vi "HFRR ADV v05.vi"() -> ()   [LabVIEW 2025] (continued)
                n2416 = Wait (ms)(milliseconds to wait=u32 200) -> ()  [unwired: 1 out]
              }
            }
            n2417 = local read "Com Port 3"() -> (w3502:refnum<visa-resource-name>)
            n2418 = local read "Humidity Str Rec"() -> (w3504:string)
            n2419 = Not Equal?(x="Set Rh", y=w3526) -> (x != y?=w3531:bool)
            n2420 = Number To Decimal String(number="Set Rh") -> (decimal integer string=w3529:string)  [unwired: 1 in]
            n2421 = Not Equal?(x=w3502, y=w3501) -> (x != y?=w3497:bool)
            n2422 = Concatenate Strings("#setPoint00" ("string"), w3529) -> (w3530:string)
            n2423 = case shown="False" w3531 {
              tunnel: w3530 -> [_ w3550]
              frame False {
                n2424 = local read "Humidity"() -> (w3547:bool)
                n2425 = case shown="True" w3547 {
                  frame False {
                    n2426 = local write "Humidity Str Send"("stop" ("Humidity Str Send")) -> ()
                  }
                  frame True {
                    n2427 = local write "Humidity Str Send"("start" ("Humidity Str Send")) -> ()
                  }
                }
              }
              frame True {
                n2428 = local write "Humidity Str Send"(w3550) -> ()
              }
            }
            n2429 = Or(x=w3497, y="Re-Initialise") -> (x .or. y?=w3496:bool)
            n2430 = String Subset(string=w3504, offset (0)=7) -> (substring=w3519:string)  [unwired: 1 in]
            n2431 = Match Pattern(string=w3504, regular expression="?") -> (offset past match=w3522:i32)  [unwired: 1 in, 3 out]
            n2432 = Match Pattern(string=w3504, regular expression="v") -> (offset past match=w3525:i32)  [unwired: 1 in, 3 out]
            n2433 = case shown="True" w3496 {
              tunnel: w3499 -> [w3536 _]
              tunnel: [w3536 errorcluster {"status"=TRUE, "code"=0, "source"="Init"} ("error out")] -> w3498
              frame False {
              }
              frame True {
              }
            }
            n2434 = Equal?(x=w3522, y=-1) -> (x = y?=w3506:bool)
            n2435 = Match Pattern(string=w3519, regular expression="g") -> (after substring=w3520:string, offset past match=w3511:i32)  [unwired: 1 in, 2 out]
            n2436 = Match Pattern(string=w3519, regular expression="y") -> (after substring=w3518:string, offset past match=w3512:i32)  [unwired: 1 in, 2 out]
            n2437 = Greater?(x=w3512, y=w3511) -> (0:w3517:bool)
            n2438 = Greater Or Equal To 0?(x=w3512) -> (x >= 0?=w3509:bool)
            n2439 = Greater Or Equal To 0?(x=w3511) -> (x >= 0?=w3510:bool)
            n2440 = Or(x=w3509, y=w3510) -> (x .or. y?=w3508:bool)
            n2441 = Greater Or Equal To 0?(x=w3525) -> (x >= 0?=w3507:bool)
            n2442 = Select(t=w3518, s=w3517, f=w3520) -> (s? t:f=w3513:string)
            n2443 = case shown="Error" w3498 {
              selector: w3498 -> [w3563 w3609]
              tunnel: [w3561 w3602] -> w3535
              tunnel: w3501 -> [w3564 w3608]
              tunnel: [w3562 w3611] -> w3534
              tunnel: w3532 -> [w3551 w3610]
              tunnel: [w3558 w3610] -> w3533
              frame No Error {
                n2444 = call "Elapsed Time7"() -> ("Time has Elapsed"=w3557:bool)  [unwired: 12 in, 7 out]
                n2445 = Not Equal?(x="Humidity Str Send", y=w3551) -> (x != y?=w3553:bool)
                n2446 = Or(x=w3553, y=w3557) -> (x .or. y?=w3556:bool)
                n2447 = Select(t="Humidity Str Send", s=w3553, f="vals" ("regular expression")) -> (s? t:f=w3552:string)
                n2448 = Or(x=w3556, y="Send") -> (x .or. y?=w3560:bool)
                n2449 = case shown="True" w3560 {
                  tunnel: [w3567 w3572] -> w3561
                  tunnel: w3564 -> [w3566 w3580]
                  tunnel: w3563 -> [w3567 w3579]
                  tunnel: [w3566 w3573] -> w3562
                  tunnel: w3552 -> [_ w3578]
                  tunnel: [w3565 w3569] -> w3558
                  tunnel: "Humidity Str Send" -> [_ w3570]
                  tunnel: w3553 -> [_ w3571]
                  tunnel: w3551 -> [w3565 w3568]
                  frame False {
                  }
                  frame True {
                    n2450 = flat-sequence {
                      tunnel: w3580 -> [w3588]
                      tunnel: w3579 -> [w3587]
                      tunnel: w3578 -> [w3584]
                      tunnel: [w3586] -> w3577
                      tunnel: [w3585] -> w3576
                      tunnel: w3577 -> [w3591]
                      tunnel: w3576 -> [w3590]
                      tunnel: [w3591] -> w3575
                      tunnel: [w3590] -> w3574
                      tunnel: w3575 -> [w3598]
                      tunnel: w3574 -> [w3597]
                      tunnel: [w3596] -> w3573
                      tunnel: [w3595] -> w3572
                      frame #0 {
                        n2451 = local write "Ser Led"(TRUE ("Boolean 4")) -> ()
                        n2452 = Concatenate Strings(w3584, "\r") -> (w3583:string)
                        n2453 = VISA Write(VISA resource name=w3588, write buffer=w3583, error in (no error)=w3587) -> (VISA resource name out=w3586:refnum<visa-resource-name>, error out=w3585:errorcluster)  [unwired: 1 out]
                      }
                      frame #1 {
                        n2454 = Wait (ms)(milliseconds to wait="wait") -> ()  [unwired: 1 out]
                      }
                      frame #2 {
                        w3593 = FALSE ("Send")
                        n2455 = property class="Instr"(reference=w3598, error in=w3597) -> (reference out=w3599:refnum<visa-resource-name>, error out=w3600:errorcluster, "Serial Settings:Number of Bytes at Serial Port"=w3592:u32)
                        "Humidity 2" <- w3592
                        n2456 = local write "Send"(w3593) -> ()
                        n2457 = local write "Ser Led"(w3593) -> ()
                        n2458 = VISA Read(VISA resource name=w3599, byte count=w3592, error in (no error)=w3600) -> (VISA resource name out=w3596:refnum<visa-resource-name>, read buffer=→"Humidity Str Rec":string, error out=w3595:errorcluster)  [unwired: 1 out]
                      }
                    }
                    n2459 = Select(t=w3570, s=w3571, f=w3568) -> (s? t:f=w3569:string)
                  }
                }
              }
              frame Error {
                w3616 = u16 0 items=["None"=0, "XON/XOFF"=1, "RTS/CTS"=2, "DTR/DSR"=4] ("flow control")
                w3612 = u16 0 items=["None", "Odd", "Even", "Mark", "Space"] ("parity")
                w3615 = u16 10 items=["1.0"=10, "1.5"=15, "2.0"=20] ("stop bits")
                n2460 = VISA Close(VISA resource name=w3608, error in (no error)=w3609) -> (error out=w3607:errorcluster)
                n2461 = local write "humid"("" ("humid")) -> ()
                n2462 = local write "Humidity Str Rec"("" ("Humidity Str Rec")) -> ()
                n2463 = call <vilib>:"Clear Errors.vi"("error in (no error)"=w3607) -> ("error out"=w3606:errorcluster)  [unwired: 5 in, 1 out]
                n2464 = local read "Com Port 3"() -> (w3605:refnum<visa-resource-name>)
                n2465 = call-poly "VISA Configure Serial Port"("VISA resource name"=w3605, "timeout (10sec)"=u32 1000, "termination char\n(0xA = '\\n' = LF)"=u8 10 ("termination char\n(0xA = '\\n' = LF)"), "Enable Termination\nChar (T)"=FALSE ("Enable Termination Char (T)"), "baud rate (9600)"="Humidity BaudRate", "data bits (8)"=u16 8 ("data bits"), "parity (0:none)"=w3612, "error in (no error)"=w3606, "stop bits (10: 1 bit)"=w3615, "flow control (0:none)"=w3616) -> ("VISA resource name out"=w3611:refnum<visa-resource-name>, "error out"=w3602:errorcluster)  [unwired: 4 in]
              }
            }
            n2466 = Compound Arithmetic op=AND(w3507, w3506, w3508) -> (w3505:bool)
            n2467 = case shown="True" w3505 {
              tunnel: w3504 -> [_ _]
              tunnel: w3513 -> [_ w3543]
              frame False {
              }
              frame True {
                w3541 = " " ("regular expression")
                n2468 = Match Pattern(string=w3543, regular expression=" ") -> (after substring=w3545:string)  [unwired: 1 in, 3 out]
                n2469 = Match Pattern(string=w3545, regular expression=w3541) -> (before substring=→"humid":string, after substring=w3542:string)  [unwired: 1 in, 2 out]
                n2470 = Match Pattern(string=w3542, regular expression=w3541) -> (before substring=→"temp_@Rh sensor":string)  [unwired: 1 in, 3 out]
              }
            }
            n2471 = local read "Quit"() -> (w3494:bool)
          }
          n2472 = VISA Close(VISA resource name=w3490, error in (no error)=w3491) -> (error out=w3487:errorcluster)
          n2473 = call <vilib>:"Clear Errors.vi"("error in (no error)"=w3487) -> ()  [unwired: 5 in, 2 out]
        }
        frame Enabled {
        }
      }
    }
    frame Enabled {
    }
  }
  n2474 = while {
    tunnel: [w3624] -> _
    i -> [w3624]
    stop <- w3619 stop-if-true
    # "Langauage selection"
    n2475 = property on="FF Calibration g" class="WFGraph (strict)"("Plot Area:Colors:FG Color"=u32 0) -> ()  [unwired: 2 in, 2 out]
    n2476 = Equal?(x="Lan flag", y=22.0) -> ()  [unwired: 1 out]
    n2477 = disable-structure shown="Disabled" {
      frame Disabled {
        n2478 = stacked-sequence {
          frame #0 {
            n2479 = case shown="\"Russian\"" "Language Selection" {
              tunnel: [0 1] -> w3626
              frame "English", Default {
              }
              frame "Russian" {
              }
            }
            n2480 = for {
              N: 130 -> [_]
              tunnel: "Table" -> [w3635]
              tunnel: w3626 -> [w3634]
              i -> [w3633]
              n2481 = Index Array(array=w3635, index (row)=w3633, index (col)=w3634) -> (element=w3632:string)
              n2482 = case shown="7" w3633 {
                tunnel: w3632 -> [w3636 w3637 _ w3638 w3639 w3640 w3641 w3642 w3643 w3644 w3645 w3646 w3647 w3648 w3649 w3650 w3651 w3652 w3653 w3654 w3655 w3656 w3657 w3658 w3659 w3660 w3661 w3662 w3663 _ _ w3664 w3665 w3666 w3667 w3668 w3669 w3678 w3685 w3692 w3699 w3703 w3706 w3709 w3711 w3713 w3714 w3715 w3716 w3717 w3718 w3719 w3720 w3721 w3722 w3723 w3724 w3725 w3726 w3727 w3728 w3729 w3730 w3731 w3732 w3733 w3734 w3735 w3736 w3737 w3738 w3739 w3740 w3741 w3742 w3743 w3744 w3745 w3746 w3747 w3748 w3749 w3750 w3751 w3752 w3753 w3754 w3755 w3756 w3757 w3758 w3759 w3760 w3761 w3762 w3763 w3764 w3765 w3766 w3767 w3768 w3769 w3770 w3771 w3772 _ w3773 w3774 w3775 w3776 w3777 w3778 w3779 w3780 w3781 w3782 w3783 w3784 w3785 _ w3786 w3787 w3788 w3789 w3790 w3791 _]
                frame 0 {
                  n2483 = local write "S"(w3636) -> ()
                }
                frame 1 {
                  n2484 = local write "S 2"(w3637) -> ()
                }
                frame 2 {
                }
                frame 3 {
                  n2485 = local write "S 4"(w3638) -> ()
                }
                frame 4 {
                  n2486 = property on="FILE" class="Str"("Caption.Text"=w3639) -> ()  [unwired: 2 in, 2 out]
                }
                frame 5 {
                  n2487 = property on="Fuel Discription :" class="Str"("Caption.Text"=w3640) -> ()  [unwired: 2 in, 2 out]
                }
                frame 6 {
                  n2488 = property on="Remarks :" class="Str"("Caption.Text"=w3641) -> ()  [unwired: 2 in, 2 out]
                }
                frame 7 {
                  n2489 = property on="Save & Continue" class="Bool (strict)"("Boolean Text.Text"=w3642) -> ()  [unwired: 2 in, 2 out]
                }
                frame 8 {
                }
                frame 9 {
                  n2490 = property on="Set Hz" class="DigNum (strict)"("Caption.Text"=w3644) -> ()  [unwired: 2 in, 2 out]
                }
                frame 10 {
                  "String 3" <- w3645
                }
                frame 11 {
                  n2491 = property on="NORMAL LOAD" class="DigNum (strict)"("Caption.Text"=w3646) -> ()  [unwired: 2 in, 2 out]
                }
                frame 12 {
                  "String 5" <- w3647
                }
                frame 13 {
                  n2492 = property on="Set Temp" class="DigNum (strict)"("Caption.Text"=w3648) -> ()  [unwired: 2 in, 2 out]
                }
                frame 14 {
                  n2493 = local write "S 15"(w3649) -> ()
                }
                frame 15 {
                  n2494 = property on="Set Rh" class="DigNum (strict)"("Caption.Text"=w3650) -> ()  [unwired: 2 in, 2 out]
                }
                frame 16 {
                  "String 13" <- w3651
                  "String 26" <- w3651
                }
                frame 17 {
                  n2495 = local write "S 18"(w3652) -> ()
                }
                frame 18 {
                  "String 17" <- w3653
                }
                frame 19 {
                  n2496 = property on="test time" class="DigNum (strict)"("Caption.Text"=w3654) -> ()  [unwired: 2 in, 2 out]
                }
                frame 20 {
                  "String 18" <- w3655
                  "String 22" <- w3655
                }
                frame 21 {
                  n2497 = property on="Elapsed time" class="DigNum (strict)"("Caption.Text"=w3656) -> ()  [unwired: 2 in, 2 out]
                }
                frame 22 {
                  n2498 = property on="Samplingtime 2" class="DigNum (strict)"("Caption.Text"=w3657) -> ()  [unwired: 2 in, 2 out]
                }
                frame 23 {
                  "String 21" <- w3658
                }
                frame 24 {
                  n2499 = property on="Countdown" class="DigNum (strict)"("Caption.Text"=w3659) -> ()  [unwired: 2 in, 2 out]
                }
                frame 25 {
                  n2500 = property on="Countdown 2" class="DigNum (strict)"("Caption.Text"=w3660) -> ()  [unwired: 2 in, 2 out]
                }
                frame 26 {
                  n2501 = property on="Engage" class="Bool (strict)"("Boolean Text.Text"=w3661) -> ()  [unwired: 2 in, 2 out]
                }
                frame 27 {
                  n2502 = property on="Boolean  4" class="Bool (strict)"("Boolean Text.Text"=w3662) -> ()  [unwired: 2 in, 2 out]
                }
                frame 28 {
                  n2503 = property on="Test \nStatus" class="Bool (strict)"("Boolean Text.Text"=w3663) -> ()  [unwired: 2 in, 2 out]
                }
                frame 29 {
                }
                frame 30 {
                }
                frame 31 {
                  n2504 = property on="FF Calibration g" class="WFGraph (strict)"("X Scale.Name Label.Text"=w3664) -> ()  [unwired: 2 in, 2 out]
                }
                frame 32 {
                  n2505 = property on="RSTCOF" class="Bool"("Boolean Text.Text"=w3665) -> ()  [unwired: 2 in, 2 out]
                  n2506 = property on="RST FF" class="Bool"("Boolean Text.Text"=w3665) -> ()  [unwired: 2 in, 2 out]
                  n2507 = property on="RST TEMP" class="Bool"("Boolean Text.Text"=w3665) -> ()  [unwired: 2 in, 2 out]
                  n2508 = property on="RSTV1 3" class="Bool"("Boolean Text.Text"=w3665) -> ()  [unwired: 2 in, 2 out]
                  n2509 = property on="rstv2" class="Bool"("Boolean Text.Text"=w3665) -> ()  [unwired: 2 in, 2 out]
                  n2510 = property on="RSTV1 2" class="Bool"("Boolean Text.Text"=w3665) -> ()  [unwired: 2 in, 2 out]
                  n2511 = property on="RST CP" class="Bool"("Boolean Text.Text"=w3665) -> ()  [unwired: 2 in, 2 out]
                }
                frame 33 {
                  "S 61" <- w3666
                }
                frame 34 {
                  "String 23" <- w3667
                }
                frame 35 {
                  n2512 = property on="Rh Before" class="DigNum (strict)"("Caption.Text"=w3668) -> ()  [unwired: 2 in, 2 out]
                }
                frame 36 {
                  n2513 = Match Pattern(string=w3669, regular expression=",") -> (before substring=→"bs":string, after substring=→"as":string)  [unwired: 1 in, 2 out]
                  n2514 = property on="Rh After" class="DigNum (strict)"("Caption.Text"=w3669) -> ()  [unwired: 2 in, 2 out]
                }
                frame 37 {
                  n2515 = Match Pattern(string=w3678, regular expression=",") -> (before substring=w3677:string, after substring=w3676:string)  [unwired: 1 in, 2 out]
                  "bs" <- w3677
                  "as" <- w3676
                  n2516 = Concatenate Strings(w3677, w3676) -> (w3673:string)
                  n2517 = property on="Humidity before test 2" class="DigNum (strict)"("Caption.Text"=w3673) -> ()  [unwired: 2 in, 2 out]
                  n2518 = property on="Humidity before test" class="DigNum (strict)"("Caption.Text"=w3673) -> ()  [unwired: 2 in, 2 out]
                  n2519 = Concatenate Strings(w3673, "=" ("string")) -> (w3674:string)
                  n2520 = local write "S 38"(w3674) -> ()
                }
                frame 38 {
                  n2521 = Match Pattern(string=w3685, regular expression=",") -> (before substring=w3684:string, after substring=w3683:string)  [unwired: 1 in, 2 out]
                  "bs" <- w3684
                  "as" <- w3683
                  n2522 = Concatenate Strings(w3684, w3683) -> (w3680:string)
                  n2523 = property on="Humidity after test 2" class="DigNum (strict)"("Caption.Text"=w3680) -> ()  [unwired: 2 in, 2 out]
                  n2524 = Concatenate Strings(w3680, "=" ("string")) -> (w3682:string)
                  n2525 = property on="Humidity after test" class="DigNum (strict)"("Caption.Text"=w3680) -> ()  [unwired: 2 in, 2 out]
                  n2526 = local write "S 39"(w3682) -> ()
                }
                frame 39 {
                  n2527 = Match Pattern(string=w3692, regular expression=",") -> (before substring=w3691:string, after substring=w3690:string)  [unwired: 1 in, 2 out]
                  "bs" <- w3691
                  "as" <- w3690
                  n2528 = Concatenate Strings(w3691, w3690) -> (w3687:string)
                  n2529 = property on="Temperature before test 2" class="DigNum (strict)"("Caption.Text"=w3687) -> ()  [unwired: 2 in, 2 out]
                  n2530 = property on="Temperature before test" class="DigNum (strict)"("Caption.Text"=w3687) -> ()  [unwired: 2 in, 2 out]
                  n2531 = Concatenate Strings(w3687, "=" ("string")) -> (→"String 34":string)
                }
                frame 40 {
                  n2532 = Match Pattern(string=w3699, regular expression=",") -> (before substring=w3698:string, after substring=w3697:string)  [unwired: 1 in, 2 out]
                  "bs" <- w3698
                  "as" <- w3697
                  n2533 = Concatenate Strings(w3698, w3697) -> (w3694:string)
                  n2534 = property on="Temperature after test 2" class="DigNum (strict)"("Caption.Text"=w3694) -> ()  [unwired: 2 in, 2 out]
                  n2535 = Concatenate Strings(w3694, "=" ("string")) -> (→"String 35":string)
                  n2536 = property on="Temperature after test" class="DigNum (strict)"("Caption.Text"=w3694) -> ()  [unwired: 2 in, 2 out]
                }
                frame 41 {
                  n2537 = property on="AVP" class="DigNum (strict)"("Caption.Text"=w3703) -> ()  [unwired: 2 in, 2 out]
                  n2538 = property on="AVP 2" class="DigNum (strict)"("Caption.Text"=w3703) -> ()  [unwired: 2 in, 2 out]
                  n2539 = Concatenate Strings(w3703, "=" ("string")) -> (→"String 36":string)
                }
                frame 42 {
                  n2540 = property on="MWSD" class="DigNum (strict)"("Caption.Text"=w3706) -> ()  [unwired: 2 in, 2 out]
                  n2541 = property on="MWSD 2" class="DigNum (strict)"("Caption.Text"=w3706) -> ()  [unwired: 2 in, 2 out]
                  n2542 = Concatenate Strings(w3706, "=" ("string")) -> (→"String 37":string)
                }
                frame 43 {
                  n2543 = property on="HCF 2" class="DigNum (strict)"("Caption.Text"=w3709) -> ()  [unwired: 2 in, 2 out]
                  n2544 = property on="HCF" class="DigNum (strict)"("Caption.Text"=w3709) -> ()  [unwired: 2 in, 2 out]
                  n2545 = Concatenate Strings(w3709, "=" ("string")) -> (→"String 38":string)
                }
                frame 44 {
                  n2546 = Concatenate Strings(w3711, "=" ("string")) -> (→"String 39":string)
                  n2547 = property on="WS1.4 2" class="DigNum (strict)"("Caption.Text"=w3711) -> ()  [unwired: 2 in, 2 out]
                  n2548 = property on="WS1.4" class="DigNum (strict)"("Caption.Text"=w3711) -> ()  [unwired: 2 in, 2 out]
                }
                frame 45 {
                  n2549 = property on="Save Results" class="Bool (strict)"("Boolean Text.Text"=w3713) -> ()  [unwired: 2 in, 2 out]
                }
                frame 46 {
                  n2550 = local write "S 47"(w3714) -> ()
                }
                frame 47 {
                  n2551 = local write "S 48"(w3715) -> ()
                }
                frame 48 {
                  n2552 = local write "S 49"(w3716) -> ()
                }
                frame 49 {
                  n2553 = local write "S 50"(w3717) -> ()
                }
                frame 50 {
                  n2554 = local write "S 51"(w3718) -> ()
                }
                frame 51 {
                  n2555 = local write "S 52"(w3719) -> ()
                }
                frame 52 {
                  n2556 = local write "S 53"(w3720) -> ()
                }
                frame 53 {
                  n2557 = local write "S 54"(w3721) -> ()
                }
                frame 54 {
                  n2558 = local write "S 55"(w3722) -> ()
                }
                frame 55 {
                  n2559 = local write "S 56"(w3723) -> ()
                }
                frame 56 {
                  n2560 = local write "S 57"(w3724) -> ()
                }
                frame 57 {
                  n2561 = local write "S 58"(w3725) -> ()
                }
                frame 58 {
                  n2562 = local write "S 59"(w3726) -> ()
                }
                frame 59 {
                  n2563 = local write "S 60"(w3727) -> ()
                }
                frame 60 {
                  n2564 = local write "S 62"(w3728) -> ()
                }
                frame 61 {
                  n2565 = local write "S 63"(w3729) -> ()
                }
                frame 62 {
                  n2566 = local write "S 64"(w3730) -> ()
                }
                frame 63 {
                  n2567 = local write "S 65"(w3731) -> ()
                }
                frame 64 {
                  n2568 = local write "S 66"(w3732) -> ()
                }
                frame 65 {
                  n2569 = local write "S 67"(w3733) -> ()
                }
                frame 66 {
                  n2570 = local write "S 68"(w3734) -> ()
                }
                frame 67 {
                  n2571 = local write "S 69"(w3735) -> ()
                }
                frame 68 {
                  n2572 = local write "S 70"(w3736) -> ()
                }
                frame 69 {
                  n2573 = local write "S 71"(w3737) -> ()
                }
                frame 70 {
                  n2574 = local write "S 72"(w3738) -> ()
                }
                frame 71 {
                  n2575 = local write "S 73"(w3739) -> ()
                }
                frame 72 {
                  n2576 = local write "S 74"(w3740) -> ()
                }
                frame 73 {
                  n2577 = local write "S 75"(w3741) -> ()
                }
                frame 74 {
                  n2578 = local write "S 76"(w3742) -> ()
                }
                frame 75 {
                  n2579 = local write "S 77"(w3743) -> ()
                }
                frame 76 {
                  n2580 = local write "S 78"(w3744) -> ()
                }
                frame 77 {
                  n2581 = local write "S 79"(w3745) -> ()
                }
                frame 79 {
                  n2582 = property on="Sample Temperature" class="XYGraph (strict)"("Y Scale.Name Label.Text"=w3746) -> ()  [unwired: 2 in, 2 out]
                }
                frame 80 {
                  n2583 = local write "S 81"(w3747) -> ()
                  n2584 = property on="Humidity" class="XYGraph (strict)"("Y Scale.Name Label.Text"=w3747) -> ()  [unwired: 2 in, 2 out]
                }
                frame 78 {
                  n2585 = property on="Air Temperature" class="XYGraph (strict)"("X Scale.Name Label.Text"=w3748) -> ()  [unwired: 2 in, 2 out]
                  n2586 = property on="Humidity" class="XYGraph (strict)"("X Scale.Name Label.Text"=w3748) -> ()  [unwired: 2 in, 2 out]
                  n2587 = property on="Sample Temperature" class="XYGraph (strict)"("X Scale.Name Label.Text"=w3748) -> ()  [unwired: 2 in, 2 out]
                  n2588 = property on="Coefficient Of Friction" class="XYGraph (strict)"("X Scale.Name Label.Text"=w3748) -> ()  [unwired: 2 in, 2 out]
                }
                frame 81 {
                  n2589 = property on="Air Temperature" class="XYGraph (strict)"("Y Scale.Name Label.Text"=w3749) -> ()  [unwired: 2 in, 2 out]
                }
                frame 82 {
                  n2590 = local write "S 84"(w3750) -> ()
                }
                frame 83 {
                  n2591 = local write "S 85"(w3751) -> ()
                }
                frame 84 {
                  n2592 = local write "S 86"(w3752) -> ()
                }
                frame 85 {
                  n2593 = local write "S 87"(w3753) -> ()
                }
                frame 86 {
                  n2594 = local write "S 88"(w3754) -> ()
                }
                frame 87 {
                  n2595 = property on="FF Calibration g" class="WFGraph (strict)"("Y Scale.Name Label.Text"=w3755) -> ()  [unwired: 2 in, 2 out]
                }
                frame 88 {
                  n2596 = local write "S 90"(w3756) -> ()
                }
                frame 89 {
                  n2597 = local write "S 91"(w3757) -> ()
                }
                frame 90 {
                  n2598 = local write "S 92"(w3758) -> ()
                }
                frame 91 {
                  n2599 = local write "S 93"(w3759) -> ()
                }
                frame 92 {
                  n2600 = local write "S 94"(w3760) -> ()
                }
                frame 93 {
                  n2601 = local write "S 95"(w3761) -> ()
                }
                frame 94 {
                  n2602 = local write "S 96"(w3762) -> ()
                }
                frame 95 {
                  n2603 = local write "S 97"(w3763) -> ()
                }
                frame 96 {
                  n2604 = local write "S 98"(w3764) -> ()
                }
                frame 97 {
                  n2605 = local write "S 99"(w3765) -> ()
                }
                frame 98 {
                  n2606 = local write "S 100"(w3766) -> ()
                }
                frame 99 {
                  n2607 = local write "S 101"(w3767) -> ()
                }
                frame 100 {
                  n2608 = local write "S 102"(w3768) -> ()
                }
                frame 101 {
                  n2609 = local write "S 103"(w3769) -> ()
                }
                frame 102 {
                  n2610 = local write "S 104"(w3770) -> ()
                }
                frame 103 {
                  n2611 = local write "S 105"(w3771) -> ()
                }
                frame 104 {
                  n2612 = local write "S 106"(w3772) -> ()
                }
                frame 105 {
                }
                frame 106 {
                  n2613 = property on="OK Button 17" class="Bool (strict)"("Boolean Text.Text"=w3773) -> ()  [unwired: 2 in, 2 out]
                }
                frame 107 {
                  n2614 = property on="OK Button 16" class="Bool (strict)"("Boolean Text.Text"=w3774) -> ()  [unwired: 2 in, 2 out]
                }
                frame 108 {
                  n2615 = property on="TITTLE" class="Str"("Caption.Text"=w3775) -> ()  [unwired: 2 in, 2 out]
                }
                frame 109 {
                  "String 30" <- w3776
                }
                frame 110 {
                  n2616 = property on="Test Date" class="Str"("Caption.Text"=w3777) -> ()  [unwired: 2 in, 2 out]
                  "String 31" <- w3777
                }
                frame 111 {
                  n2617 = property on="Sample ID" class="Str"("Caption.Text"=w3778) -> ()  [unwired: 2 in, 2 out]
                  "String 32" <- w3778
                }
                frame 112 {
                  n2618 = property on="Tested by" class="Str"("Caption.Text"=w3779) -> ()  [unwired: 2 in, 2 out]
                  "String 33" <- w3779
                }
                frame 113 {
                  n2619 = property on="System Configured Printers 2" class="Arr (strict)"("Caption.Text"=w3780) -> ()  [unwired: 2 in, 2 out]
                }
                frame 114 {
                  n2620 = property on="Selected Printer" class="Str"("Caption.Text"=w3781) -> ()  [unwired: 2 in, 2 out]
                }
                frame 115 {
                  n2621 = property on="Select Printer 3" class="DigNum (strict)"("Caption.Text"=w3782) -> ()  [unwired: 2 in, 2 out]
                }
                frame 116 {
                  n2622 = property on="Print" class="Bool (strict)"("Boolean Text.Text"=w3783) -> ()  [unwired: 2 in, 2 out]
                }
                frame 117 {
                  "String 41" <- w3784
                }
                frame 118 {
                  n2623 = property on="tested by" class="Str"("Caption.Text"=w3785) -> ()  [unwired: 2 in, 2 out]
                }
                frame 119 {
                }
                frame 120 {
                  n2624 = property on="Export" class="Bool (strict)"("Boolean Text.Text"=w3786) -> ()  [unwired: 2 in, 2 out]
                }
                frame 121 {
                  n2625 = property on="TEMP INTERCEPT:" class="DigNum (strict)"("Caption.Text"=w3787) -> ()  [unwired: 2 in, 2 out]
                }
                frame 122 {
                  n2626 = property on="AIR TEMP INTERCEPT:" class="DigNum (strict)"("Caption.Text"=w3788) -> ()  [unwired: 2 in, 2 out]
                }
                frame 123 {
                  n2627 = property on="Select File Type" class="Enum (strict)"("Caption.Text"=w3789) -> ()  [unwired: 2 in, 2 out]
                }
                frame 124 {
                  n2628 = property on="s.NO" class="Str"("Caption.Text"=w3790) -> ()  [unwired: 2 in, 2 out]
                  "String 45" <- w3790
                }
                frame 125 {
                  n2629 = property on="trip1 8" class="Bool (strict)"("Boolean Text.Text"=w3791) -> ()  [unwired: 2 in, 2 out]
                }
                frame 126, Default {
                }
              }
            }
          }
          frame #1 {
            w3799 = TRUE ("Visible")
            n2630 = local read "S 91"() -> (w3816:string)
            n2631 = local read "S 90"() -> (w3815:string)
            n2632 = local read "S 88"() -> (w3814:string)
            n2633 = property on="Threshold" class="DigNum (strict)"("Caption.Text"=w3816) -> ()  [unwired: 2 in, 2 out]
            n2634 = property on="File Path" class="Path"("Caption.Text"=w3815) -> ()  [unwired: 2 in, 2 out]
            n2635 = property on="SrvM CP" class="Bool (strict)"("Boolean Text.Text"=w3814) -> ()  [unwired: 2 in, 2 out]
            n2636 = local read "S 71"() -> (w3809:string)
            n2637 = local read "S 86"() -> (w3811:string)
            n2638 = local read "S 85"() -> (w3812:string)
            n2639 = local read "S 87"() -> (w3810:string)
            n2640 = local read "S 84"() -> (w3813:string)
            n2641 = local read "S 103"() -> (w3798:string)
            n2642 = local read "S 104"() -> (w3797:string)
            n2643 = property on="ENTER THE NEW PASSWORD" class="Str"("Caption.Text"=w3810) -> ()  [unwired: 2 in, 2 out]
            n2644 = property on="Password" class="Str"("Caption.Text"=w3812) -> ()  [unwired: 2 in, 2 out]
            n2645 = property on="ENTER CURRENT PASSWORD" class="Str"("Caption.Text"=w3811) -> ()  [unwired: 2 in, 2 out]
            n2646 = property on="EDIT" class="Bool (strict)"("Boolean Text.Text"=w3809) -> ()  [unwired: 2 in, 2 out]
            n2647 = property on="SAVE" class="Bool (strict)"("Boolean Text.Text"=w3813) -> ()  [unwired: 2 in, 2 out]
            n2648 = Build Array(w3798, w3797) -> (w3796:string[])
            n2649 = property on="Heater Button" class="Bool (strict)"("Strings [4]"=w3796) -> ()  [unwired: 2 in, 2 out]
            n2650 = property on="CH-HUMIDITY WET" class="DigNum (strict)"("Caption.Size to Text?"=w3799) -> ()  [unwired: 2 in, 2 out]
            n2651 = property on="CH-HUMIDITY DRY" class="DigNum (strict)"("Caption.Size to Text?"=w3799) -> ()  [unwired: 2 in, 2 out]
            n2652 = property on="CH-POWER -" class="DigNum (strict)"("Caption.Size to Text?"=w3799) -> ()  [unwired: 2 in, 2 out]
            n2653 = property on="CH-HEATER" class="DigNum (strict)"("Caption.Size to Text?"=w3799) -> ()  [unwired: 2 in, 2 out]
            n2654 = property on="CH-POWER +" class="DigNum (strict)"("Caption.Size to Text?"=w3799) -> ()  [unwired: 2 in, 2 out]
            n2655 = local read "S 92"() -> (w3808:string)
            n2656 = local read "S 93"() -> (w3807:string)
            n2657 = local read "S 105"() -> (w3794:string)
            n2658 = local read "S 106"() -> (w3793:string)
            n2659 = Build Array(w3808, w3807) -> ()  [unwired: 1 out]
            n2660 = Build Array(w3794, w3793) -> (w3795:string[])
            n2661 = local read "S 95"() -> (w3805:string)
            n2662 = local read "S 94"() -> (w3806:string)
            n2663 = local read "bs"() -> (w3821:string)
            n2664 = local read "as"() -> (w3822:string)
            n2665 = property on="Humidity" class="Bool (strict)"("Strings [4]"=w3795) -> ()  [unwired: 2 in, 2 out]
            n2666 = Concatenate Strings(w3821, "\r", w3822) -> ()  [unwired: 1 out]
            n2667 = property on="STROKE GAIN :" class="DigNum (strict)"("Caption.Text"=w3805) -> ()  [unwired: 2 in, 2 out]
            n2668 = property on="DISPLACEMENT :" class="DigNum (strict)"("Caption.Text"=w3806) -> ()  [unwired: 2 in, 2 out]
            n2669 = property on="Rh After" class="DigNum (strict)"("Caption.Size to Text?"=TRUE ("Caption.Size to Text")) -> ()  [unwired: 2 in, 2 out]
            n2670 = local read "S 48"() -> (w3845:string)
            n2671 = local read "S 50"() -> (w3843:string)
            n2672 = local read "S 51"() -> (w3842:string)
            n2673 = local read "S 49"() -> (w3844:string)
            n2674 = local read "S 52"() -> (w3841:string)
            n2675 = local read "as"() -> (w3826:string)
            n2676 = local read "bs"() -> (w3827:string)
            n2677 = local read "S 56"() -> (w3840:string)
            n2678 = local read "S 57"() -> (w3839:string)
            n2679 = local read "S 58"() -> (w3838:string)
            n2680 = local read "S 59"() -> (w3837:string)
            n2681 = property on="OPEN" class="Bool (strict)"("Boolean Text.Text"=w3841) -> ()  [unwired: 2 in, 2 out]
            n2682 = property on="OPEN 1" class="Bool (strict)"("Boolean Text.Text"=w3845) -> ()  [unwired: 2 in, 2 out]
            n2683 = property on="OPEN 2" class="Bool (strict)"("Boolean Text.Text"=w3844) -> ()  [unwired: 2 in, 2 out]
            n2684 = property on="OPEN 3" class="Bool (strict)"("Boolean Text.Text"=w3843) -> ()  [unwired: 2 in, 2 out]
            n2685 = property on="OPEN 4" class="Bool (strict)"("Boolean Text.Text"=w3842) -> ()  [unwired: 2 in, 2 out]
            n2686 = Concatenate Strings(w3827, "\r", w3826) -> ()  [unwired: 1 out]
            n2687 = local read "S 102"() -> (w3800:string)
            n2688 = property on="КОФ1" class="DigNum (strict)"("Caption.Text"=w3840) -> ()  [unwired: 2 in, 2 out]
            n2689 = local read "S 98"() -> (w3804:string)
            n2690 = local read "S 99"() -> (w3803:string)
            n2691 = local read "S 100"() -> (w3802:string)
            n2692 = local read "S 101"() -> (w3801:string)
            n2693 = property on="КОФ2" class="DigNum (strict)"("Caption.Text"=w3839) -> ()  [unwired: 2 in, 2 out]
            n2694 = property on="КОФ3" class="DigNum (strict)"("Caption.Text"=w3838) -> ()  [unwired: 2 in, 2 out]
            n2695 = property on="КОФ4" class="DigNum (strict)"("Caption.Text"=w3837) -> ()  [unwired: 2 in, 2 out]
            n2696 = local read "bs"() -> (w3825:string)
            n2697 = local read "as"() -> (w3824:string)
            n2698 = property on="CH-POWER +" class="DigNum (strict)"("Caption.Text"=w3804) -> ()  [unwired: 2 in, 2 out]
            n2699 = property on="CH-POWER -" class="DigNum (strict)"("Caption.Text"=w3803) -> ()  [unwired: 2 in, 2 out]
            n2700 = property on="CH-HEATER" class="DigNum (strict)"("Caption.Text"=w3802) -> ()  [unwired: 2 in, 2 out]
            n2701 = property on="CH-HUMIDITY DRY" class="DigNum (strict)"("Caption.Text"=w3801) -> ()  [unwired: 2 in, 2 out]
            n2702 = property on="CH-HUMIDITY WET" class="DigNum (strict)"("Caption.Text"=w3800) -> ()  [unwired: 2 in, 2 out]
            n2703 = local read "S 60"() -> (w3836:string)
            n2704 = local read "S 54"() -> (w3846:string)
            n2705 = Concatenate Strings(w3825, "\r", w3824) -> ()  [unwired: 1 out]
            n2706 = Concatenate Strings(w3846, w3836) -> ()  [unwired: 1 out]
            n2707 = local read "S 77"() -> (→"String 43":string)
            n2708 = local read "S 76"() -> (w3819:string)
            n2709 = local read "S 78"() -> (w3818:string)
            n2710 = local read "S 71"() -> (w3830:string)
            n2711 = local read "S 66"() -> (w3835:string)
            n2712 = local read "S 67"() -> (w3834:string)
            n2713 = local read "S 68"() -> (w3833:string)
            n2714 = local read "S 69"() -> (w3832:string)
            n2715 = local read "S 70"() -> (w3831:string)
            n2716 = property on="AIR TEMP" class="DigNum (strict)"("Caption.Text"=w3818) -> ()  [unwired: 2 in, 2 out]
            n2717 = property on="Set Strk" class="DigNum (strict)"("Caption.Text"=w3819) -> ()  [unwired: 2 in, 2 out]
            n2718 = property on="FRIC. FORCE :" class="DigNum (strict)"("Caption.Text"=w3835) -> ()  [unwired: 2 in, 2 out]
            n2719 = property on="TEMPERATURE :" class="DigNum (strict)"("Caption.Text"=w3834) -> ()  [unwired: 2 in, 2 out]
            n2720 = property on="SPEED OUT:" class="DigNum (strict)"("Caption.Text"=w3833) -> ()  [unwired: 2 in, 2 out]
            n2721 = property on="AIR TEMPERATURE :" class="DigNum (strict)"("Caption.Text"=w3832) -> ()  [unwired: 2 in, 2 out]
            n2722 = property on="HUMIDITY:" class="DigNum (strict)"("Caption.Text"=w3831) -> ()  [unwired: 2 in, 2 out]
            n2723 = property on="EDIT" class="Bool (strict)"("Boolean Text.Text"=w3830) -> ()  [unwired: 2 in, 2 out]
            n2724 = local read "S 79"() -> (w3817:string)
            n2725 = property on="Stroke" class="DigNum (strict)"("Caption.Text"=w3817) -> ()  [unwired: 2 in, 2 out]
          }
          frame #2 {
          }
        }
        n2726 = local write "Lan flag"(10.0 ("Lan flag")) -> ()
      }
      frame Enabled {
      }
    }
    n2727 = Wait (ms)(milliseconds to wait=u32 2000) -> ()  [unwired: 1 out]
    n2728 = local read "Quit"() -> (w3619:bool)
  }
  n2729 = disable-structure shown="Disabled" {
    frame Disabled {
      n2730 = while {
        tunnel: [w3848] -> _
        i -> [w3848]
        stop <- w3847 continue-if-true
        n2731 = Wait (ms)(milliseconds to wait=u32 50) -> ()  [unwired: 1 out]
        n2732 = stacked-sequence {
          frame #0 {
            # "Controls Text color"
            # "Controls BG color"
            n2733 = property on="FILE" class="Str"("Text.Text Colors:Text Color"="SC  Text") -> ()  [unwired: 2 in, 2 out]
            n2734 = property on="Fuel Discription :" class="Str"("Text.Text Colors:Text Color"="SC  Text") -> ()  [unwired: 2 in, 2 out]
            n2735 = property on="tested by" class="Str"("Text.Text Colors:Text Color"="SC  Text") -> ()  [unwired: 2 in, 2 out]
            n2736 = property on="Remarks :" class="Str"("Text.Text Colors:Text Color"="SC  Text") -> ()  [unwired: 2 in, 2 out]
            n2737 = property class="DigNum (strict)"("Numeric Text.Text Colors:BG Color"="NC BG") -> ()  [unwired: 2 in, 2 out]
            n2738 = property class="DigNum (strict)"("Numeric Text.Text Colors:BG Color"="NC BG") -> ()  [unwired: 2 in, 2 out]
            n2739 = property class="DigNum (strict)"("Numeric Text.Text Colors:BG Color"="NC BG") -> ()  [unwired: 2 in, 2 out]
            n2740 = property class="DigNum (strict)"("Numeric Text.Text Colors:BG Color"="NC BG") -> ()  [unwired: 2 in, 2 out]
            n2741 = property class="DigNum (strict)"("Numeric Text.Text Colors:BG Color"="NC BG") -> ()  [unwired: 2 in, 2 out]
            n2742 = property class="DigNum (strict)"("Numeric Text.Text Colors:BG Color"="NC BG") -> ()  [unwired: 2 in, 2 out]
            n2743 = property class="DigNum (strict)"("Numeric Text.Text Colors:BG Color"="NC BG") -> ()  [unwired: 2 in, 2 out]
            n2744 = property class="DigNum (strict)"("Numeric Text.Text Colors:BG Color"="NC BG") -> ()  [unwired: 2 in, 2 out]
            n2745 = property class="DigNum (strict)"("Numeric Text.Text Colors:BG Color"="NC BG") -> ()  [unwired: 2 in, 2 out]
            n2746 = property class="DigNum (strict)"("Numeric Text.Text Colors:BG Color"="NC BG") -> ()  [unwired: 2 in, 2 out]
            n2747 = property class="DigNum (strict)"("Numeric Text.Text Colors:BG Color"="NC BG") -> ()  [unwired: 2 in, 2 out]
            n2748 = property class="DigNum (strict)"("Numeric Text.Text Colors:BG Color"="NC BG") -> ()  [unwired: 2 in, 2 out]
            n2749 = property on="FILE" class="Str"("Text.Text Colors:BG Color"="SC BG 3") -> ()  [unwired: 2 in, 2 out]
            n2750 = property on="Fuel Discription :" class="Str"("Text.Text Colors:BG Color"="SC BG 3") -> ()  [unwired: 2 in, 2 out]
            n2751 = property on="tested by" class="Str"("Text.Text Colors:BG Color"="SC BG 3") -> ()  [unwired: 2 in, 2 out]
            n2752 = property on="Remarks :" class="Str"("Text.Text Colors:BG Color"="SC BG 3") -> ()  [unwired: 2 in, 2 out]
            n2753 = property class="DigNum (strict)"("Numeric Text.Text Colors:Text Color"="NC Text") -> ()  [unwired: 2 in, 2 out]
            n2754 = property class="DigNum (strict)"("Numeric Text.Text Colors:Text Color"="NC Text") -> ()  [unwired: 2 in, 2 out]
            n2755 = property class="DigNum (strict)"("Numeric Text.Text Colors:Text Color"="NC Text") -> ()  [unwired: 2 in, 2 out]
            n2756 = property class="DigNum (strict)"("Numeric Text.Text Colors:Text Color"="NC Text") -> ()  [unwired: 2 in, 2 out]
            n2757 = property class="DigNum (strict)"("Numeric Text.Text Colors:Text Color"="NC Text") -> ()  [unwired: 2 in, 2 out]
            n2758 = property class="DigNum (strict)"("Numeric Text.Text Colors:Text Color"="NC Text") -> ()  [unwired: 2 in, 2 out]
            n2759 = property class="DigNum (strict)"("Numeric Text.Text Colors:Text Color"="NC Text") -> ()  [unwired: 2 in, 2 out]
            n2760 = property class="DigNum (strict)"("Numeric Text.Text Colors:Text Color"="NC Text") -> ()  [unwired: 2 in, 2 out]
            n2761 = property class="DigNum (strict)"("Numeric Text.Text Colors:Text Color"="NC Text") -> ()  [unwired: 2 in, 2 out]
            n2762 = property class="DigNum (strict)"("Numeric Text.Text Colors:Text Color"="NC Text") -> ()  [unwired: 2 in, 2 out]
            n2763 = property class="DigNum (strict)"("Numeric Text.Text Colors:Text Color"="NC Text") -> ()  [unwired: 2 in, 2 out]
            n2764 = property class="DigNum (strict)"("Numeric Text.Text Colors:Text Color"="NC Text") -> ()  [unwired: 2 in, 2 out]
            n2765 = property class="DigNum (strict)"("Numeric Text.Text Colors:Text Color"="NI Text  2") -> ()  [unwired: 2 in, 2 out]
            n2766 = property class="DigNum (strict)"("Numeric Text.Text Colors:Text Color"="NI Text  2") -> ()  [unwired: 2 in, 2 out]
            n2767 = property class="DigNum (strict)"("Numeric Text.Text Colors:Text Color"="NI Text  2") -> ()  [unwired: 2 in, 2 out]
            n2768 = property class="DigNum (strict)"("Numeric Text.Text Colors:Text Color"="NI Text  2") -> ()  [unwired: 2 in, 2 out]
            n2769 = property class="DigNum (strict)"("Numeric Text.Text Colors:Text Color"="NI Text  2") -> ()  [unwired: 2 in, 2 out]
            n2770 = property class="DigNum (strict)"("Numeric Text.Text Colors:Text Color"="NI Text  2") -> ()  [unwired: 2 in, 2 out]
            n2771 = property class="DigNum (strict)"("Numeric Text.Text Colors:Text Color"="NI Text  2") -> ()  [unwired: 2 in, 2 out]
            n2772 = property class="DigNum (strict)"("Numeric Text.Text Colors:Text Color"="NI Text  2") -> ()  [unwired: 2 in, 2 out]
            n2773 = property class="DigNum (strict)"("Numeric Text.Text Colors:Text Color"="NI Text  2") -> ()  [unwired: 2 in, 2 out]
            n2774 = property class="DigNum (strict)"("Numeric Text.Text Colors:Text Color"="NI Text  2") -> ()  [unwired: 2 in, 2 out]
            n2775 = property class="DigNum (strict)"("Numeric Text.Text Colors:Text Color"="NI Text  2") -> ()  [unwired: 2 in, 2 out]
            n2776 = property class="DigNum (strict)"("Numeric Text.Text Colors:Text Color"="NI Text  2") -> ()  [unwired: 2 in, 2 out]
            n2777 = property class="DigNum (strict)"("Numeric Text.Text Colors:Text Color"="NI Text  2") -> ()  [unwired: 2 in, 2 out]
            n2778 = property class="DigNum (strict)"("Numeric Text.Text Colors:Text Color"="NI Text  2") -> ()  [unwired: 2 in, 2 out]
            n2779 = property class="DigNum (strict)"("Numeric Text.Text Colors:Text Color"="NI Text  2") -> ()  [unwired: 2 in, 2 out]
            n2780 = property class="DigNum (strict)"("Numeric Text.Text Colors:Text Color"="NI Text  2") -> ()  [unwired: 2 in, 2 out]
            n2781 = property on="Coefficient Of Friction" class="XYGraph (strict)"("Plot Area:Colors:FG Color"="GFG  2", "Plot Area:Colors:BG Color"="GBG   2") -> ()  [unwired: 2 in, 2 out]
            n2782 = property on="Humidity" class="XYGraph (strict)"("Plot Area:Colors:FG Color"="GFG  2", "Plot Area:Colors:BG Color"="GBG   2") -> ()  [unwired: 2 in, 2 out]
            n2783 = property on="Air Temperature" class="XYGraph (strict)"("Plot Area:Colors:FG Color"="GFG  2", "Plot Area:Colors:BG Color"="GBG   2") -> ()  [unwired: 2 in, 2 out]
            n2784 = property on="Sample Temperature" class="XYGraph (strict)"("Plot Area:Colors:FG Color"="GFG  2", "Plot Area:Colors:BG Color"="GBG   2") -> ()  [unwired: 2 in, 2 out]
            n2785 = property class="DigNum (strict)"("Numeric Text.Text Colors:BG Color"="NI BG 2") -> ()  [unwired: 2 in, 2 out]
            n2786 = property class="DigNum (strict)"("Numeric Text.Text Colors:BG Color"="NI BG 2") -> ()  [unwired: 2 in, 2 out]
            n2787 = property class="DigNum (strict)"("Numeric Text.Text Colors:BG Color"="NI BG 2") -> ()  [unwired: 2 in, 2 out]
            n2788 = property class="DigNum (strict)"("Numeric Text.Text Colors:BG Color"="NI BG 2") -> ()  [unwired: 2 in, 2 out]
            n2789 = property class="DigNum (strict)"("Numeric Text.Text Colors:BG Color"="NI BG 2") -> ()  [unwired: 2 in, 2 out]
            n2790 = property class="DigNum (strict)"("Numeric Text.Text Colors:BG Color"="NI BG 2") -> ()  [unwired: 2 in, 2 out]
            n2791 = property class="DigNum (strict)"("Numeric Text.Text Colors:BG Color"="NI BG 2") -> ()  [unwired: 2 in, 2 out]
            n2792 = property class="DigNum (strict)"("Numeric Text.Text Colors:BG Color"="NI BG 2") -> ()  [unwired: 2 in, 2 out]
            n2793 = property class="DigNum (strict)"("Numeric Text.Text Colors:BG Color"="NI BG 2") -> ()  [unwired: 2 in, 2 out]
            n2794 = property class="DigNum (strict)"("Numeric Text.Text Colors:BG Color"="NI BG 2") -> ()  [unwired: 2 in, 2 out]
            n2795 = property class="DigNum (strict)"("Numeric Text.Text Colors:BG Color"="NI BG 2") -> ()  [unwired: 2 in, 2 out]
            n2796 = property class="DigNum (strict)"("Numeric Text.Text Colors:BG Color"="NI BG 2") -> ()  [unwired: 2 in, 2 out]
            n2797 = property class="DigNum (strict)"("Numeric Text.Text Colors:BG Color"="NI BG 2") -> ()  [unwired: 2 in, 2 out]
            n2798 = property class="DigNum (strict)"("Numeric Text.Text Colors:BG Color"="NI BG 2") -> ()  [unwired: 2 in, 2 out]
            n2799 = property class="DigNum (strict)"("Numeric Text.Text Colors:BG Color"="NI BG 2") -> ()  [unwired: 2 in, 2 out]
            n2800 = property class="DigNum (strict)"("Numeric Text.Text Colors:BG Color"="NI BG 2") -> ()  [unwired: 2 in, 2 out]
            n2801 = property class="Bool"("Colors [4]"="Boolean BC T & BG") -> ()  [unwired: 2 in, 2 out]
            n2802 = property on="Save & Continue" class="Bool (strict)"("Colors [4]"="Boolean BC T & BG") -> ()  [unwired: 2 in, 2 out]
            n2803 = property on="Heater Button" class="Bool (strict)"("Colors [4]"="Boolean BC T & BG") -> ()  [unwired: 2 in, 2 out]
            n2804 = property class="Bool"("Colors [4]"="Boolean BC T & BG") -> ()  [unwired: 2 in, 2 out]
            n2805 = property on="Humidity" class="Bool (strict)"("Colors [4]"="Boolean BC T & BG") -> ()  [unwired: 2 in, 2 out]
            n2806 = property class="Bool (strict)"("Colors [4]"="Boolean BC T & BG") -> ()  [unwired: 2 in, 2 out]
            n2807 = property on="RUN" class="Bool (strict)"("Colors [4]"="Boolean BC T & BG") -> ()  [unwired: 2 in, 2 out]
            n2808 = property on="trip1 8" class="Bool (strict)"("Colors [4]"="Boolean BC T & BG") -> ()  [unwired: 2 in, 2 out]
            n2809 = property class="Bool"("Colors [4]"="Boolean BC T & BG") -> ()  [unwired: 2 in, 2 out]
            n2810 = property class="Bool (strict)"("Colors [4]"="Boolean BC T & BG") -> ()  [unwired: 2 in, 2 out]
            n2811 = property on="OPEN 1" class="Bool (strict)"("Colors [4]"="Boolean BC T & BG 2") -> ()  [unwired: 2 in, 2 out]
            n2812 = property on="OPEN 2" class="Bool (strict)"("Colors [4]"="Boolean BC T & BG 2") -> ()  [unwired: 2 in, 2 out]
            n2813 = property on="OPEN 3" class="Bool (strict)"("Colors [4]"="Boolean BC T & BG 2") -> ()  [unwired: 2 in, 2 out]
            n2814 = property on="OPEN 4" class="Bool (strict)"("Colors [4]"="Boolean BC T & BG 2") -> ()  [unwired: 2 in, 2 out]
            n2815 = property on="OPEN" class="Bool (strict)"("Colors [4]"="Boolean BC T & BG 2") -> ()  [unwired: 2 in, 2 out]
            n2816 = property on="rstv2" class="Bool"("Colors [4]"="Boolean BC T & BG 2") -> ()  [unwired: 2 in, 2 out]
            n2817 = property on="RST CP" class="Bool"("Colors [4]"="Boolean BC T & BG 2") -> ()  [unwired: 2 in, 2 out]
            n2818 = property on="RSTV1 3" class="Bool"("Colors [4]"="Boolean BC T & BG 2") -> ()  [unwired: 2 in, 2 out]
            n2819 = property on="RSTV1 2" class="Bool"("Colors [4]"="Boolean BC T & BG 2") -> ()  [unwired: 2 in, 2 out]
          }
          frame #1 {
          }
        }
        n2820 = local read "Quit"() -> (w3847:bool)
      }
    }
    frame Enabled {
    }
  }
  n2821 = while {
    shift-right: [w3865] -> _
    shift-left: _ -> [w3866]
    shift-right: [w3863] -> _
    shift-left: T13 {"Read Heave and Surge"="", "Bytes at Heave Port"=0.0, "Heave and Surge COM Port:"="COM9", "Com Port 2"="COM7", "Residual Due"="", "Heave COM Status 2"=TRUE, "Heave COM Status"=TRUE, "Port 2"=TRUE, "Sway PPR"=6400.0, "Surge PPR"=6400.0, "Heave PPR"=6400.0, "Sway Pitch"=2.0, "Surge Pitch"=3.0, "Heave Pitch"=4.0, "Sway Pulses/mm"=320.0, "Surge Pulses/mm"=1600.0, "Heave Pulses/mm"=1600.0, "inner loop"=0.0, "Read Heave and Surge 2"="", "String 36"="", "Write S"=FALSE, "WriteCC1"=[""], "Heave COM Loop"=0, "LastCom"="", "EXIT"=FALSE, "Error Heave"={"status"=TRUE, "code"=-1073807343, "source"=""}} -> [w3862]
    shift-right: [w3860] -> _
    shift-left: enum16{"init", "MAIN", "Panel Close"}."init" -> [w3861]
    stop <- w3864 stop-if-true
    n2822 = case shown="\"MAIN\"" w3861 {
      tunnel: w3866 -> [w3880 w3895 w3965 w3967]
      tunnel: [w3874 w3913 w3965 w3967] -> w3865
      tunnel: [_ _ TRUE _] -> w3864
      tunnel: [w3870 w3910 w3963 w3966] -> w3863
      tunnel: w3862 -> [w3877 w3894 w3963 w3966]
      tunnel: [enum16{"init", "MAIN", "Panel Close"}."MAIN" w3888 _ _] -> w3860
      frame "init" {
        n2823 = Bundle By Name(cluster=w3877, "Heave and Surge COM Port:"="Humidity") -> (w3876:T13)
        n2824 = call "Instrument fgv.vi"("Enum"=T19."INIT", "error in (no error) 2"=w3880, "INPUT"=w3876) -> ("error"=w3878:errorcluster, "output"=w3873:T13)  [unwired: 6 in, 1 out]
        n2825 = case shown="Error" w3878 {
          selector: w3878 -> [w3882 _]
          tunnel: [w3882 w3886] -> w3874
          tunnel: w3873 -> [w3881 w3884]
          tunnel: [w3881 w3883] -> w3871
          frame No Error {
          }
          frame Error {
            n2826 = call "Instrument fgv.vi"("Enum"=T19."ERROR INIT", "INPUT"=w3884) -> ("error"=w3887:errorcluster, "output"=w3883:T13)  [unwired: 7 in, 1 out]
            n2827 = call <vilib>:"Clear Errors.vi"("error in (no error)"=w3887) -> ("error out"=w3886:errorcluster)  [unwired: 5 in, 1 out]
          }
        }
        n2828 = local read "LastCom"() -> (w3869:string)
        n2829 = Unbundle By Name(w3871) -> ("Heave COM Status 2"=→"Heave COM Status 2" →"Instrument Status":bool, "Error Heave"=→"Error Heave":errorcluster)  [unwired: 1 out]
        n2830 = Bundle By Name(cluster=w3871, "LastCom"=w3869) -> (w3870:T13)
      }
      frame "MAIN" {
        (unwired) u32 10 ("milliseconds to wait")
        n2831 = Unbundle By Name(w3894) -> ("Com Port 2"=w3915:refnum<visa-resource-name>)
        n2832 = local write "Com Port 4"(w3915) -> ()
        n2833 = local read "Humidity"() -> (w3892:refnum<visa-resource-name>)
        n2834 = Divide(x="Heave PPR", y="Heave Pitch") -> (x/y=→"Heave Pulses/mm":dbl)
        n2835 = Bundle By Name(cluster=w3894, "Heave and Surge COM Port:"=w3892) -> (w3893:T13)
        n2836 = Equal?(x=w3915, y=w3892) -> (x = y?=w3914:bool)
        n2837 = Divide(x="Sway PPR", y="Sway Pitch") -> (x/y=→"Sway Pulses/mm":dbl)
        n2838 = case shown="True" w3914 {
          tunnel: [w3919 w3936] -> w3913
          tunnel: w3895 -> [w3920 w3942]
          tunnel: w3893 -> [w3918 w3940]
          tunnel: [w3917 w3935] -> w3910
          frame False {
            n2839 = call <vilib>:"Clear Errors.vi"("error in (no error)"=w3920) -> ("error out"=w3916:errorcluster)  [unwired: 5 in, 1 out]
            n2840 = call "Instrument fgv.vi"("Enum"=T19."ERROR INIT", "error in (no error) 2"=w3916, "INPUT"=w3918) -> ("error"=w3922:errorcluster, "output"=w3917:T13)  [unwired: 6 in, 1 out]
            n2841 = call <vilib>:"Clear Errors.vi"("error in (no error)"=w3922) -> ("error out"=w3919:errorcluster)  [unwired: 5 in, 1 out]
          }
          frame True {
